vi "Simple Calibration.vi"() -> ()   [LabVIEW 2014]
doc: "This example builds a local coordinate system based on the information returned by an X-Y-Theta positioning system. The example finds the location of the template in the image and transforms the coordinates from the image coordinate system to the local system using the IMAQ Convert Pixel to Real World VI."
uses:
  <vilib>/vision/NI_Vision_Development_Module.lvlib
panel:
  out "Board Mounting Hole Location":T1 {"Image Axis (pixels)"."Y" format="%.2f"; "Image Axis (pixels)"."X" format="%.2f"}
  out "Calibration Axis":T2={"Origin Point (pixels)"={"X"=0.0, "Y"=0.0}, "Angle (degrees)"=0.0, "Axis Reference"=1} {"Axis Reference" items=["Direct", "Indirect"]; "Angle (degrees)" format="%.2f"; "Origin Point (pixels)"."Y" format="%.2f"; "Origin Point (pixels)"."X" format="%.2f"}
  in  "Delay (s.)":dbl(slide)=0.5 scale=0.0..2.0
  out "Board Corner Template":T3(plugin-control)
  out "Mounting Hole Template":T3(plugin-control)
  out "Image":T3(plugin-control)
  in  "Stop":bool
  # "Overview: Demonstrates how to use the Calibration functions to apply a simple calibration to an image, update the calibration axis as the part moves, and calculate the real world position of a feature compared with the pixel position of that same feature. \nRequirements: Vision Development Software.\nInstructions: Run the VI."
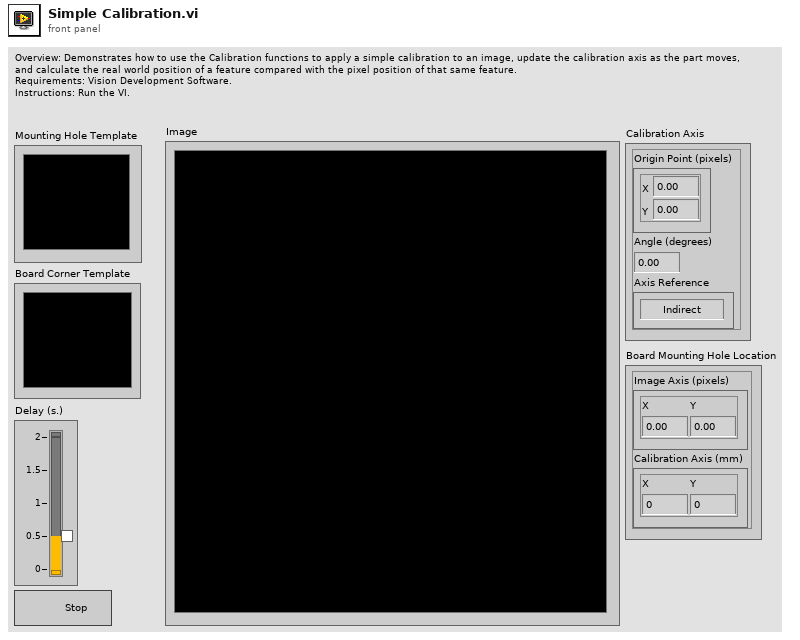
[diagram p1: front panel]
types:
  T1 = cluster{"Image Axis (pixels)":cluster{"X":dbl, "Y":dbl}, "Calibration Axis (mm)":cluster{"X":dbl, "Y":dbl}}
  T2 = cluster{"Origin Point (pixels)":cluster{"X":sgl, "Y":sgl}, "Angle (degrees)":sgl, "Axis Reference":u32}
  T3 = typedef "IMAQ Image.ctl" = refnum<image>
  T4 = typedef "Simple Grid Descriptor" = cluster{"X Step":sgl, "Y Step":sgl, "Unit":T5}
  T5 = typedef "Image Unit" = enum32{"Undefined", "Angström", "Micrometer", "Millimeter", "Centimeter", "Meter", "Kilometer", "Microinch", "Inch", "Feet", "Nautical miles", "Standard miles", "Steps"}
  T6 = typedef "Image Type" = u32
  T7 = cluster{"Position":cluster{"x":sgl, "y":sgl}, "Angle":sgl, "Scale":sgl, "Score":sgl, "Bounding Box":cluster{"x":sgl, "y":sgl}[]}[]
  T8 = cluster{"Position":cluster{"x":sgl, "y":sgl}, "Angle":sgl, "Scale":sgl, "Score":sgl, "Bounding Box":cluster{"x":sgl, "y":sgl}[]}
  T9 = cluster{"Position":cluster{"x":sgl, "y":sgl}, "Angle":sgl, "Axis Reference":u32}
  T10 = cluster{"Position":cluster{"x":sgl, "y":sgl}, "Real World Coordinates":cluster{"X":sgl, "Y":sgl}}
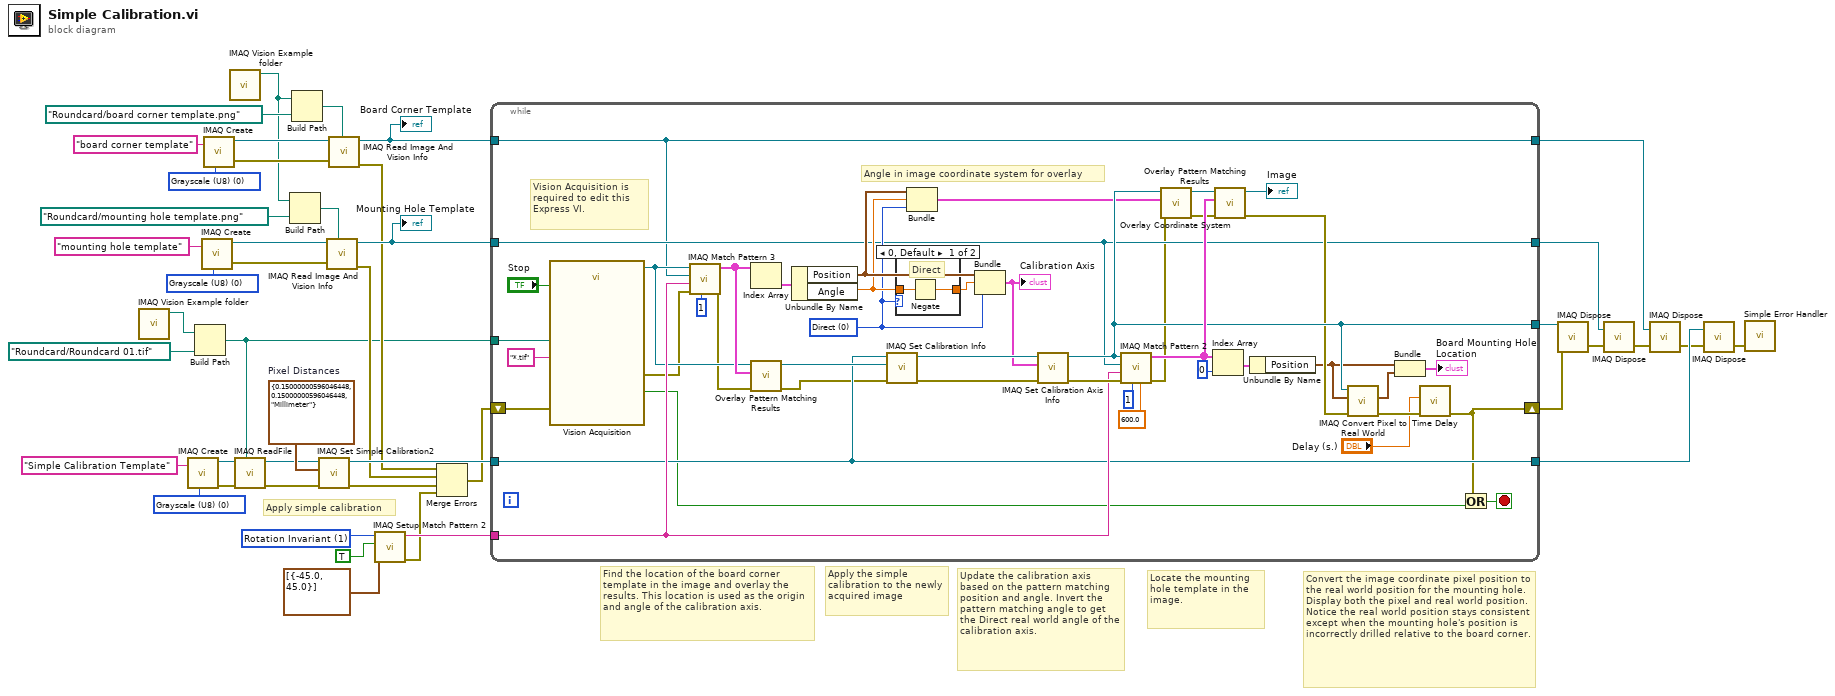
[diagram p0: block diagram]
diagram:
  w29 = u16 1 items=["Shift Invariant", "Rotation Invariant"] ("Match Mode")
  w31 = T4 {"X Step"=0.15, "Y Step"=0.15, "Unit"=enum."Millimeter"}  # Pixel Distances
  w33 = T6 0 items=["Grayscale (U8)", "Grayscale (I16)", "Grayscale (SGL)", "Complex (CSG)", "RGB (U32)", "HSL (U32)", "RGB (U64)", "Grayscale (U16)"] ("Image Type")
  w37 = T6 0 items=["Grayscale (U8)", "Grayscale (I16)", "Grayscale (SGL)", "Complex (CSG)", "RGB (U32)", "HSL (U32)", "RGB (U64)", "Grayscale (U16)"] ("Image Type")
  w38 = T6 0 items=["Grayscale (U8)", "Grayscale (I16)", "Grayscale (SGL)", "Complex (CSG)", "RGB (U32)", "HSL (U32)", "RGB (U64)", "Grayscale (U16)"] ("Image Type")
  # "Locate the mounting hole template in the image."
  # "Find the location of the board corner template in the image and overlay the results. This location is used as the origin and angle of the calibration axis."
  # "Apply the simple calibration to the newly acquired image"
  # "Update the calibration axis based on the pattern matching position and angle. Invert the pattern matching angle to get the Direct real world angle of the calibration axis."
  # "Convert the image coordinate pixel position to the real world position for the mounting hole. Display both the pixel and real world position. Notice the real world position stays consistent except when the mounting hole's position is incorrectly drilled relative to the board corner."
  # "Apply simple calibration"
  n1 = call "IMAQ Vision Example folder.vi"() -> ("Example Image Path"=w4:path)  [unwired: 11 in]
  n2 = call "IMAQ Create"("Image Name"="Simple Calibration Template", "Image Type"=w33) -> ("New Image"=w18:T3, "error out"=w11:errorcluster)  [unwired: 2 in, 1 out]
  n3 = Build Path(base path=w4, name or relative path=path "Roundcard/Roundcard 01.tif") -> (appended path=w3:path)
  n4 = call "IMAQ Create"("Image Name"="mounting hole template" ("name or relative path"), "Image Type"=w38) -> ("New Image"=w42:T3, "error out"=w43:errorcluster)  [unwired: 2 in, 1 out]
  n5 = call "IMAQ Create"("Image Name"="board corner template" ("name or relative path"), "Image Type"=w37) -> ("New Image"=w36:T3, "error out"=w35:errorcluster)  [unwired: 2 in, 1 out]
  n6 = call "IMAQ Vision Example folder.vi"() -> ("Example Image Path"=w14:path)  [unwired: 11 in]
  n7 = call "IMAQ ReadFile"("File Path"=w3, "error in (no error)"=w11, "Image"=w18) -> ("error out"=w17:errorcluster, "Image Out"=w19:T3)  [unwired: 4 in, 3 out]
  n8 = Build Path(base path=w14, name or relative path=path "Roundcard/mounting hole template.png") -> (appended path=w13:path)
  n9 = Build Path(base path=w14, name or relative path=path "Roundcard/board corner template.png") -> (appended path=w16:path)
  n10 = call "IMAQ Set Simple Calibration2"("error in (no error)"=w17, "Pixel Distances"=w31, "Image"=w19) -> ("error out"=w10:errorcluster, "Calibration Template Image"=w30:T3)  [unwired: 7 out]
  n11 = call "IMAQ Read Image And Vision Info"("File Path"=w13, "error in (no error)"=w43, "Image"=w42) -> ("error out"=w8:errorcluster, "Image Out"=w34:T3)  [unwired: 1 in, 6 out]
  "Mounting Hole Template" <- w34
  n12 = call "IMAQ Read Image And Vision Info"("File Path"=w16, "error in (no error)"=w35, "Image"=w36) -> ("error out"=w7:errorcluster, "Image Out"=w25:T3)  [unwired: 1 in, 6 out]
  "Board Corner Template" <- w25
  n13 = call "IMAQ Setup Match Pattern 2"("Rotation Angle Ranges (degrees)"=cluster{sgl, sgl}[] [{-45.0, 45.0}], "Subpixel Accuracy"=TRUE, "Match Mode"=w29) -> ("error out"=w9:errorcluster, "Match Pattern Setup Data"=w27:string)  [unwired: 2 in, 5 out]
  n14 = Merge Errors(w7, w8, w10, w9) -> (w6:errorcluster)
  n15 = while {
    tunnel: [w78] -> w40
    tunnel: w34 -> [w48]
    tunnel: w30 -> [w72]
    shift-right: [w52] -> w39
    shift-left: w6 -> [w49]
    tunnel: w27 -> [w77]
    tunnel: w25 -> [w47]
    tunnel: [w72] -> w24
    tunnel: w3 -> [w63]
    tunnel: [w48] -> w2
    tunnel: [w47] -> w1
    stop <- w50 stop-if-true
    w68 = u32 0 items=["Direct", "Indirect"] ("Axis Reference")
    # "Vision Acquisition is required to edit this Express VI."
    # "Angle in image coordinate system for overlay"
    n16 = call "Vision Acquisition"("Image Path"=w63, "Image File Type (All Types)"="*.tif" ("Pattern"), "Stop (F)"="Stop", "error in"=w49) -> ("Image Out"=w65:T3, "Stopped"=w51:bool, "error out"=w61:errorcluster)  [unwired: 21 in]
    n17 = call "IMAQ Match Pattern 3"("Number of Matches Requested"=1, "error in (no error)"=w61, "Match Pattern Setup Data"=w77, "Template Image"=w47, "Image"=w65) -> ("error out"=w60:errorcluster, "Matches"=w74:T7)  [unwired: 2 in, 3 out]
    n18 = Index Array(array=w74) -> (element=w76:T8)  [unwired: 1 in]
    n19 = call "Overlay Pattern Matching Results.vi"("error in"=w60, "Matches"=w74, "Image"=w65) -> ("error out"=w59:errorcluster, "Image Out"=w73:T3)  [unwired: 7 in]
    n20 = Unbundle By Name(w76) -> ("Position"=w71:cluster{"x":sgl, "y":sgl}, "Angle"=w70:sgl)
    n21 = call "IMAQ Set Calibration Info"("error in (no error)"=w59, "Image Dst"=w73, "Image Src"=w72) -> ("error out"=w81:errorcluster, "Calibrated Image"=w80:T3)  [unwired: 1 in, 6 out]
    n22 = case shown="0, Default" w68 {
      tunnel: w70 -> [w90 w91]
      tunnel: [w89 w91] -> w69
      frame 0, Default {
        # "Direct"
        n23 = Negate(x=w90) -> (-x=w89:sgl)
      }
      frame 1 {
        # "Indirect"
      }
    }
    n24 = Bundle("Position"=w71, "Angle"=w70, "Axis Reference"=w68) -> (w67:T9)  [unwired: 1 out]
    n25 = Bundle("Position"=w71, "Angle"=w69, "Axis Reference"=w68) -> (w66:T9)  [unwired: 1 out]
    "Calibration Axis" <- w66
    n26 = call "IMAQ Set Calibration Axis Info"("error in (no error)"=w81, "Calibration Axis Info"=w66, "Calibration Template Image In"=w80) -> ("error out"=w79:errorcluster, "Calibration Template Image Out"=w78:T3)  [unwired: 7 out]
    n27 = call "IMAQ Match Pattern 2"("Minimum Match Score"=sgl 600.0, "Number of Matches Requested"=1, "error in (no error)"=w79, "Match Pattern Setup Data"=w77, "Template Image"=w48, "Image"=w78) -> ("error out"=w46:errorcluster, "Matches"=w84:T7)  [unwired: 1 in, 3 out]
    n28 = call "Overlay Coordinate System.vi"("error in"=w46, "Calibration Axis Info"=w67, "Image"=w78) -> ("error out"=w45:errorcluster, "Image Out"=w83:T3)  [unwired: 3 in, 4 out]
    n29 = Index Array(array=w84, index=0 ("Index")) -> (element=w88:T8)
    n30 = call "Overlay Pattern Matching Results.vi"("error in"=w45, "Matches"=w84, "Image"=w83) -> ("error out"=w58:errorcluster, "Image Out"=→"Image":T3)  [unwired: 7 in]
    n31 = Unbundle By Name(w88) -> ("Position"=w57:cluster{"x":sgl, "y":sgl})
    n32 = call "IMAQ Convert Pixel to Real World"("error in (no error)"=w58, "Pixel Coordinates"=w57, "Calibrated Image"=w78) -> ("error out"=w54:errorcluster, "Real World Coordinates"=w56:cluster{"X":sgl, "Y":sgl})  [unwired: 1 in, 6 out]
    n33 = Bundle("Position"=w57, "Real World Coordinates"=w56) -> (→"Board Mounting Hole Location":T10)  [unwired: 1 in]
    n34 = call "Time Delay"("error in (no error)"=w54, "Delay Time (s)"="Delay (s.)") -> ("error out"=w52:errorcluster)  [unwired: 9 in]
    n35 = Or(x=w52, y=w51) -> (x .or. y?=w50:bool)
  }
  n36 = call "IMAQ Dispose"("Image"=w40, "error in (no error)"=w39) -> ("error out"=w41:errorcluster)  [unwired: 1 in, 3 out]
  n37 = call "IMAQ Dispose"("Image"=w2, "error in (no error)"=w41) -> ("error out"=w23:errorcluster)  [unwired: 1 in, 3 out]
  n38 = call "IMAQ Dispose"("Image"=w1, "error in (no error)"=w23) -> ("error out"=w22:errorcluster)  [unwired: 1 in, 3 out]
  n39 = call "IMAQ Dispose"("Image"=w24, "error in (no error)"=w22) -> ("error out"=w21:errorcluster)  [unwired: 1 in, 3 out]
  n40 = call <vilib>:"Simple Error Handler.vi"("error in (no error)"=w21) -> ()  [unwired: 1 in, 8 out]
